vi "Z6 - Write.vi"(8 "error in":errorcluster, 10 "Z6":i32, 11 "TSM Context Global Access in":refnum<class "TSM Context Data Access.lvclass">) -> (0 "error out":errorcluster, 3 "TSM Context Global Access out":refnum<class "TSM Context Data Access.lvclass">)   [LabVIEW 2019, in "TSM Context Data Access.lvclass"]
uses:
  TSM Context Data Access.lvclass
  TSM Context Data Access.lvclass/TSM Context Data Access.ctl
  <vilib>/NI_TestStand_SemiconductorModule/NI_TestStand_Semiconductor_Module.lvlibp
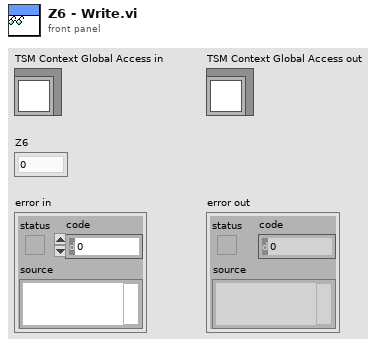
[diagram p1: front panel]
types:
  T1 = typedef "NI_TestStand_Semiconductor_Module.lvlibp/SemiconductorModuleContext.ctl" = refnum<k7>
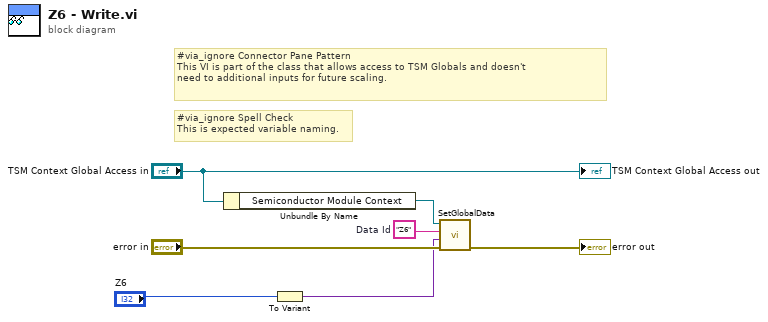
[diagram p0: block diagram]
diagram:
  w4 = "Z6"  # Data Id
  # "#via_ignore Spell Check\nThis is expected variable naming."
  # "#via_ignore Connector Pane Pattern \nThis VI is part of the class that allows access to TSM Globals and doesn't \nneed to additional inputs for future scaling."
  n1 = Unbundle By Name("TSM Context Global Access in") -> ("Semiconductor Module Context"=w5:T1)
  n2 = To Variant(anything="Z6") -> (Variant=w1:variant)
  n3 = call <vilib>:"SetGlobalData.vi"("error in (no error)"="error in", "Data"=w1, "Data Id"=w4, "Semiconductor Module Context"=w5) -> ("error out"=→"error out":errorcluster)  [unwired: 5 in, 1 out]
  "TSM Context Global Access out" <- "TSM Context Global Access in"
